vi "Get Default Config Path.vi"(8 "error in (no error)":errorcluster) -> (0 "error out":errorcluster, 3 "appended path":path)   [LabVIEW 2020, in "Process.lvclass"]
doc: "Generates the default configuration path. \nWhen called from the development environement, the default config path is the /Config relative to the project path.\nWhen called from a built exe the default config path is at C:\\Users\\<username>\\AppData\\Local\\<CompanyName>\\<ProductName> where company name and product name are the ones configured in the build specification.\nOn Linux the default config directory is \\home\\lvuser\\natinst\\bin\\config."
uses:
  Process.lvclass
  <vilib>/Utility/sysdir.llb/System Directory Type.ctl
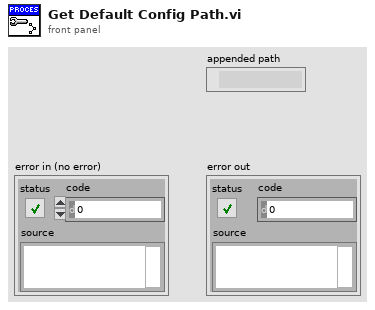
[diagram p1: front panel]
types:
  T1 = typedef "System Directory Type.ctl" = i32
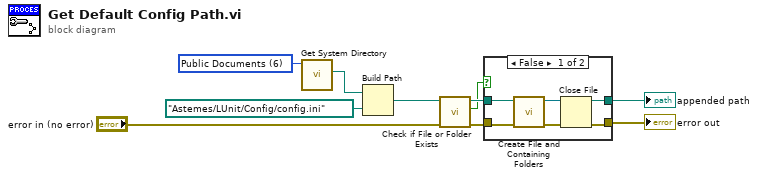
[diagram p0: block diagram]
diagram:
  w5 = T1 6 items=["User Home"=0, "User Desktop"=1, "User Documents"=2, "User Application Data"=3, "User Preferences"=4, "User Temporary"=5, "Public Documents"=6, "Public Application Data"=7, "Public Preferences"=8, "Public Cache"=13, "System Core Libraries"=9, "System Installed Libraries"=10, "Application Files"=11, "Boot Volume Root"=12] ("system directory type")
  n1 = call <vilib>:"Get System Directory.vi"("system directory type"=w5) -> ("system directory"=w7:path)  [unwired: 10 in]
  n2 = Build Path(base path=w7, name or relative path=path "Astemes/LUnit/Config/config.ini") -> (appended path=w4:path)
  n3 = call <vilib>:"Check if File or Folder Exists.vi"("error in (no error)"="error in (no error)", "path"=w4) -> ("error out"=w2:errorcluster, "file or folder exists?"=w1:bool, "dup path"=w3:path)  [unwired: 7 in]
  n4 = case shown="False" w1 {
    tunnel: [w14 w17] -> w10
    tunnel: [w13 w18] -> w8
    tunnel: w3 -> [w12 w18]
    tunnel: w2 -> [w11 w17]
    frame False {
      n5 = call <vilib>:"Create File and Containing Folders.vi"("error in (no error)"=w11, "file path"=w12) -> ("error out"=w15:errorcluster, "refnum out"=w16:refnum<file>)  [unwired: 8 in]
      n6 = Close File(refnum=w16, error in=w15) -> (path=w13:path, error out=w14:errorcluster)
    }
    frame True {
    }
  }
  "appended path" <- w8
  "error out" <- w10
